vi "配置文件断电保存(子VI).vi"   [LabVIEW 2016, in "数据传输系统.lvlib"]
uses:
  <vilib>/Utility/config.llb/NI_LVConfig.lvlib
types:
  T1 = typedef "NI_LVConfig.lvlib/Config Data RefNum.ctl" = refnum<k1>
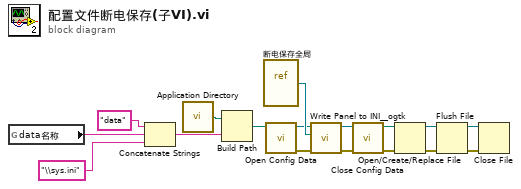
[diagram p0: block diagram]
diagram:
  n1 = global read "断电保存全局.vi" "data名称"() -> (w3:string)
  n2 = Concatenate Strings("data" ("名称或相对路径"), w3, "\\sys.ini" ("名称或相对路径")) -> (w1:string)
  n3 = call <vilib>:"Application Directory.vi"() -> ("Application Directory"=w5:path)
  n4 = Build Path(base path=w5, name or relative path=w1) -> (appended path=w6:path)
  n5 = vi-ref "断电保存全局.vi"() -> (w8:refnum<vi>)
  n6 = call <vilib>:"Open Config Data.vi"("configuration file path"=w6) -> ("error out"=w10:errorcluster, "refnum"=w7:T1)  [unwired: 8 in, 1 out]
  n7 = call <userlib>:"Write Panel to INI__ogtk.vi"("error in (no error)"=w10, "VI ref"=w8, "refnum"=w7) -> ("error out"=w11:errorcluster, "refnum out"=w9:T1)  [unwired: 7 in]
  n8 = call <vilib>:"Close Config Data.vi"("error in (no error)"=w11, "refnum"=w9) -> ("error out"=w16:errorcluster, "file path"=w17:path)  [unwired: 8 in]
  n9 = Open/Create/Replace File(file path (use dialog)=w17, error in=w16) -> (refnum out=w13:refnum<file>, error out=w12:errorcluster)  [unwired: 4 in, 1 out]
  n10 = Flush File(refnum=w13, error in=w12) -> (refnum out=w14:refnum<file>, error out=w15:errorcluster)
  n11 = Close File(refnum=w14, error in=w15) -> ()  [unwired: 2 out]
